vi "Periodic Tasks.vi"(8 "error in (no error)":errorcluster) -> ()   [LabVIEW 2013]
doc: "This VI runs in parallel to other tasks. It can contain as many user-defined periodic loops as you need. These can carry out PID or other sorts of timed response."
uses:
  PnuematicMode.ctl
  <vilib>/Rock Robotics/SystemInterfaces/Utilities/FPGA_UtilitiesLED Source.ctl
  <vilib>/Rock Robotics/SystemInterfaces/Utilities/FPGA_UtilitiesLED State.ctl
  TankDriveAction.ctl
  Example_Code/Ultrasonic/SonarAction.ctl
  AutoAlignMode.ctl
  Example_Code/Gyro/Read Angle Mode.ctl
  Robot Global Data.vi
  <vilib>/Rock Robotics/WPI/Compressor/WPI_CompressorGetSetRefNum.vi
  AutoDistance.vi
panel:
  in  "GyroBrakeScaler":dbl=1.0
  out "Finished":bool=TRUE
  in  "AccelRate":dbl
  out "HandleInputElements":i32
  out "Angle":dbl(knob) scale=0.0..360.0
  out "CurrentAngle":dbl(knob) scale=0.0..360.0
  in  "DesiredAngle":dbl format="%#_13g"
  out "CurrentDistance":dbl(slide)=255.4405658841941 scale=0.0..250.0 scale format="%3d"
  in  "Slowdown":dbl format="%#_13g"
  in  "Brake":dbl format="%#_13g"
  in  "DesiredDistance":dbl format="%#_13g"
  out "Drive loop time":u32
  out "DriveQueueElements":i32
  out "error out":errorcluster
  # "GYRO"
  # "DRIVE"
  # "AUTODISTANCE"
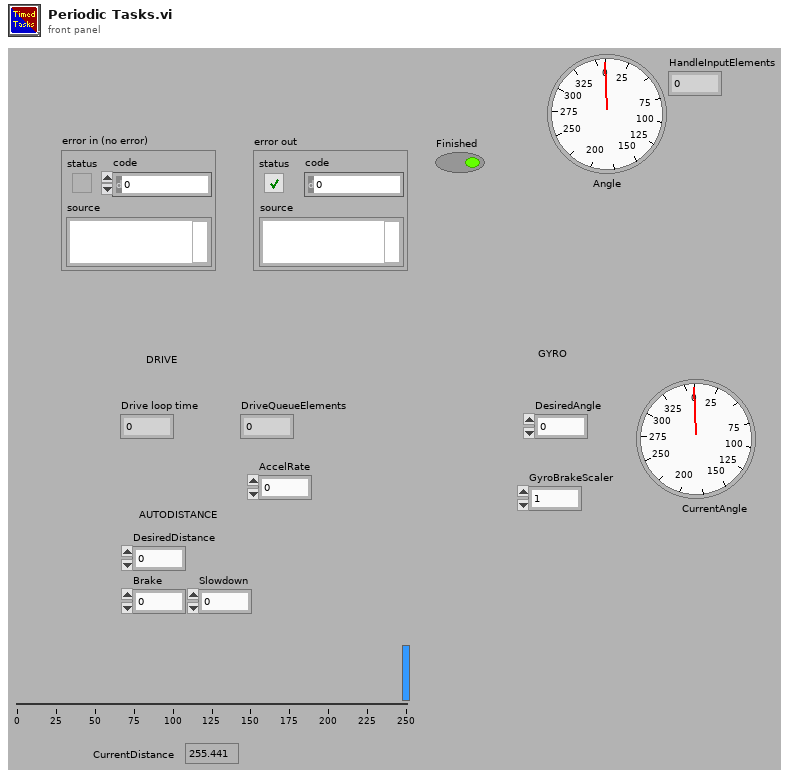
[diagram p1: front panel]
types:
  T1 = typedef "WPI_EncoderDevRef.ctl" = cluster{"DevStatus":errorcluster, "EncoderIndex":T2, "CounterIndex":T3, "DistancePerCount":dbl, "Decoding Type":T4}
  T2 = typedef "FPGA_EncoderIdx.ctl" = enum8{"Enc 0", "Enc 1", "Enc 2", "Enc 3", "Invalid"}
  T3 = typedef "FPGA_CounterCtrSystemIndex.ctl" = enum8{"Ctr 0", "Ctr 1", "Ctr 2", "Ctr 3", "Ctr 4", "Ctr 5", "Ctr 6", "Ctr 7", "Invalid"}
  T4 = typedef "WPI_EncoderType.ctl" = enum16{"1x", "2x", "4x"}
  T5 = typedef "WPI_SolenoidDevRef.ctl" = cluster{"DevStatus":errorcluster, "Solenoid Module":T6, "Forward Solenoid Channel":T7, "Reverse Solenoid Channel":T7}
  T6 = typedef "FPGA_TypedefSolenoidModule.ctl" = enum16{"Solenoid Module 1", "Solenoid Module 2"}
  T7 = typedef "WPI_SolenoidChannel.ctl" = enum8{"Solenoid 1", "Solenoid 2", "Solenoid 3", "Solenoid 4", "Solenoid 5", "Solenoid 6", "Solenoid 7", "Solenoid 8", "Invalid"}
  T8 = typedef "TankDriveAction.ctl" = enum16{"Init", "LinearDrive", "SetValue", "Disable"}
  T9 = typedef "Read Angle Mode.ctl" = enum16{"Init", "ReadAngle", "Disable"}
  T10 = typedef "SonarAction.ctl" = enum16{"Init", "ReadValue", "Disable"}
  T11 = typedef "AutoAlignMode.ctl" = enum16{"Fullspeed", "Linear"}
  T12 = typedef "DriveQueueInstruction.ctl" = cluster{"DriveInstruction":T13, "Subsystem":T14, "Action":T8, "LoopTiming":u32}
  T13 = typedef "DriveInstruction.ctl" = cluster{"cDriveLeft":dbl, "cDriveRight":dbl, "cHalfDrive":bool, "cStraightDrive":bool}
  T14 = typedef "QueueSubsystem.ctl" = enum16{"Drive", "Arm", "Catapult", "Roller"}
  T15 = typedef "TeleopInstruction.ctl" = cluster{"cDriveLeft":dbl, "cDriveRight":dbl, "cHalfDrive":bool, "cStraightDrive":bool, "cSonicShifter":bool}
  T16 = typedef "WPI_CameraDevRef.ctl" = cluster{"Camera Address":string, "CameraStatus":errorcluster, "Acquire Image Notifier":refnum<notifier>}
  T17 = typedef "PnuematicMode.ctl" = enum16{"Init", "SetState", "Disable"}
  T18 = typedef "FPGA_UtilitiesLED State.ctl" = enum16{"Off", "On", "Toggle"}
  T19 = typedef "FPGA_UtilitiesLED Source.ctl" = enum16{"User LED", "FPGA LED"}
  T20 = typedef "WPI_CompressorDevRef.ctl" = cluster{"DevStatus":errorcluster, "DigitalInputDevRef":T21, "RelayDevRef":T24}
  T21 = typedef "WPI_DigitalInputDevRef.ctl" = cluster{"DevStatus":errorcluster, "DIO Channel":T22, "Digital Module":T23}
  T22 = typedef "FPGA_DIOChannel.ctl" = enum8{"DIO 1", "DIO 2", "DIO 3", "DIO 4", "DIO 5", "DIO 6", "DIO 7", "DIO 8", "DIO 9", "DIO 10", "DIO 11", "DIO 12", "DIO 13", "DIO 14", "Invalid"}
  T23 = typedef "FPGA_TypedefDigitalModule.ctl" = enum16{"Digital Module 1", "Digital Module 2"}
  T24 = typedef "WPI_RelayDevRef.ctl" = cluster{"DevStatus":errorcluster, "Relay Channel":T25, "Digital Module":T23, "Relay Direction":T26}
  T25 = typedef "FPGA_DIORelayChannel.ctl" = enum8{"Relay 1", "Relay 2", "Relay 3", "Relay 4", "Relay 5", "Relay 6", "Relay 7", "Relay 8", "Invalid"}
  T26 = typedef "WPI_RelayDirection.ctl" = enum16{"Both directions", "Forward only", "Reverse only"}
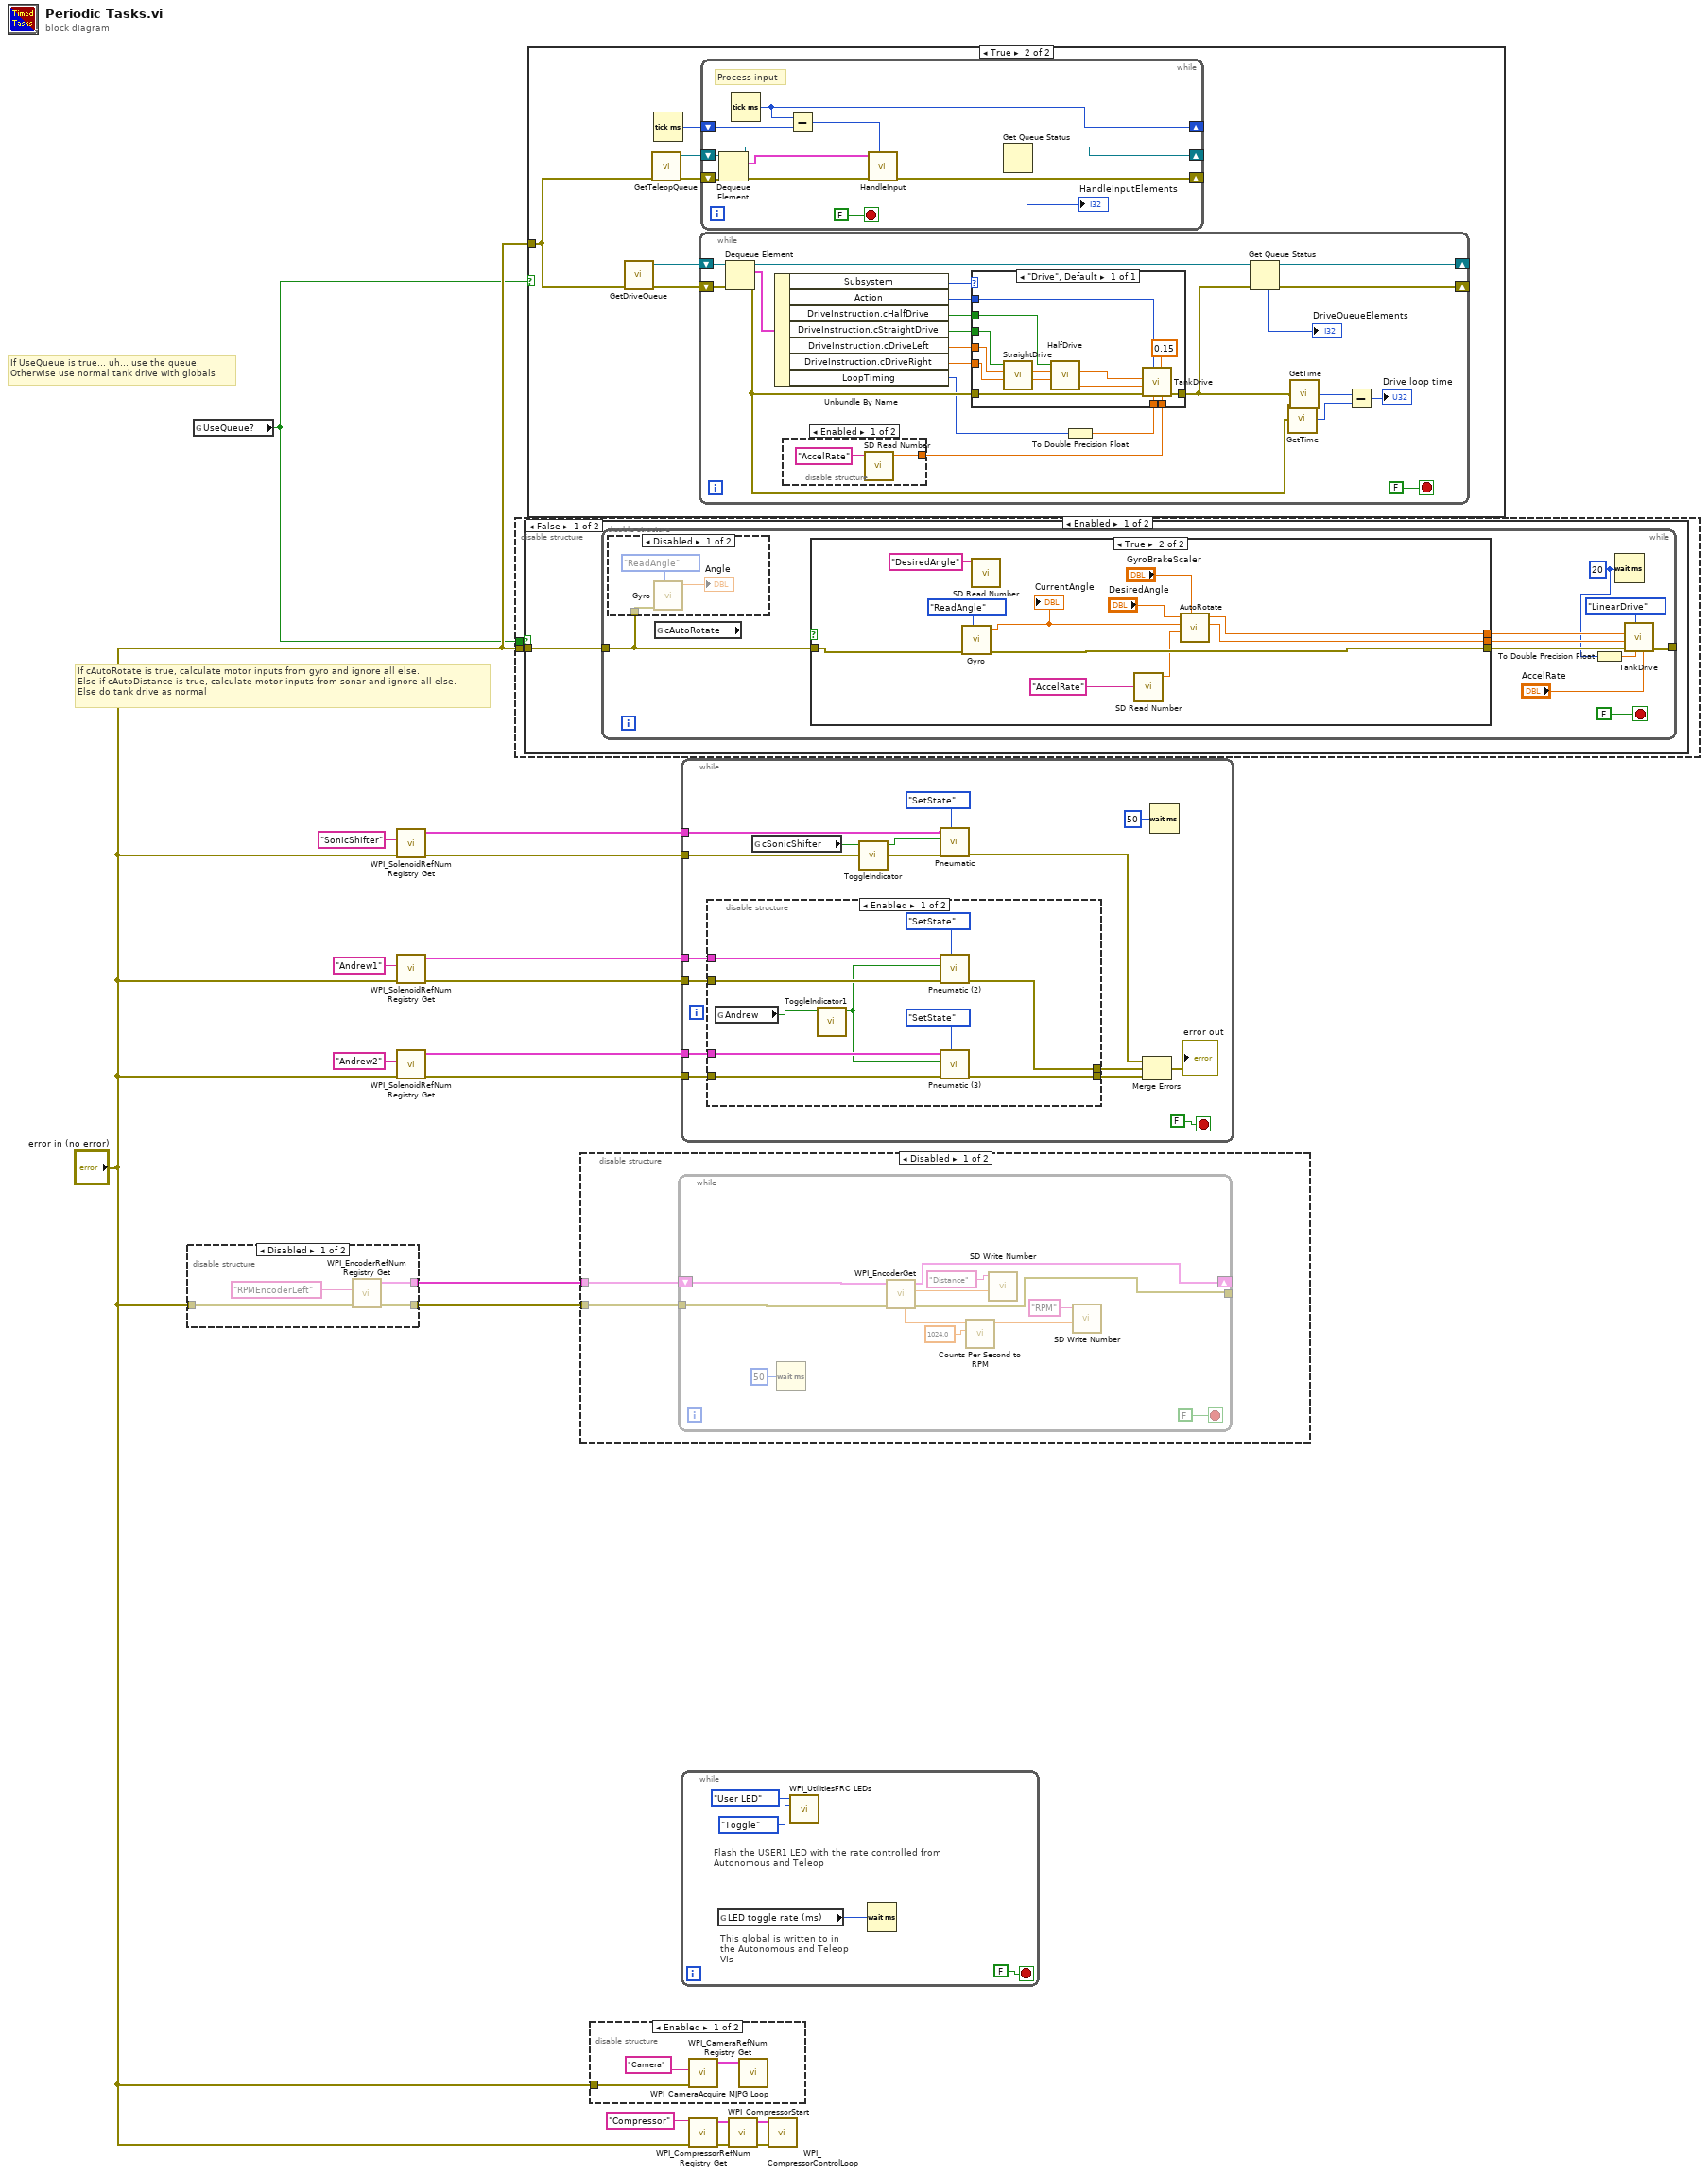
[diagram p0: block diagram]
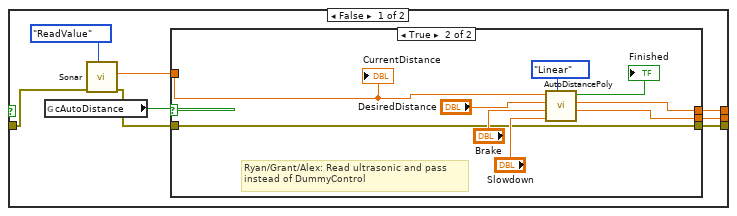
[diagram p3: hidden frame]
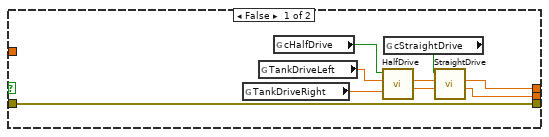
[diagram p4: hidden frame]
diagram:
  # "If UseQueue is true... uh... use the queue.\nOtherwise use normal tank drive with globals"
  # "If cAutoRotate is true, calculate motor inputs from gyro and ignore all else.\nElse if cAutoDistance is true, calculate motor inputs from sonar and ignore all else. \nElse do tank drive as normal"
  n1 = disable-structure shown="Disabled" {
    disable-tunnel: [w21 _] -> w4
    disable-tunnel: [w20 _] -> w3
    disable-tunnel: "error in (no error)" -> [w19 _]
    frame Disabled {
      n2 = call <vilib>:"WPI_EncoderRefNum Registry Get.vi"("error in (no error)"=w19, "refnum name"="RPMEncoderLeft") -> ("error out"=w20:errorcluster, "EncoderDevRef"=w21:T1)  [unwired: 8 in]
    }
    frame Enabled {
    }
  }
  n3 = global read "Robot Global Data.vi" "UseQueue?"() -> (w1:bool)
  n4 = call <vilib>:"WPI_SolenoidRefNum Registry Get.vi"("error in (no error)"="error in (no error)", "refnum name"="SonicShifter") -> ("error out"=w11:errorcluster, "SolenoidDevRef"=w13:T5)  [unwired: 8 in]
  n5 = call <vilib>:"WPI_SolenoidRefNum Registry Get.vi"("error in (no error)"="error in (no error)", "refnum name"="Andrew1") -> ("error out"=w6:errorcluster, "SolenoidDevRef"=w8:T5)  [unwired: 8 in]
  n6 = call <vilib>:"WPI_SolenoidRefNum Registry Get.vi"("error in (no error)"="error in (no error)", "refnum name"="Andrew2") -> ("error out"=w5:errorcluster, "SolenoidDevRef"=w7:T5)  [unwired: 8 in]
  n7 = disable-structure shown="Enabled" {
    disable-tunnel: "error in (no error)" -> [w24 _]
    disable-tunnel: w1 -> [w23 _]
    frame Enabled {
      n8 = case shown="False" w23 {
        tunnel: w24 -> [w25 _]
        frame False {
          n9 = while {
            tunnel: w25 -> [w32]
            tunnel: [w35] -> _
            stop <- FALSE stop-if-true
            w26 = u32 20 ("milliseconds to wait")
            n10 = disable-structure shown="Disabled" {
              disable-tunnel: w32 -> [w39 _]
              frame Disabled {
                n11 = call "Gyro.vi"("Action"=Read_Angle_Mode."ReadAngle", "error in"=w39) -> ("Angle"=→"Angle":dbl)  [unwired: 8 in, 1 out]
              }
              frame Enabled {
              }
            }
            n12 = global read "Robot Global Data.vi" "cAutoRotate"() -> (w33:bool)
            n13 = case shown="True" w33 {
              tunnel: [w47 w70] -> w30
              tunnel: [w46 w71] -> w28
              tunnel: w32 -> [w41 w73]
              tunnel: [w44 w72] -> w29
              frame False {
                n14 = global read "Robot Global Data.vi" "cAutoDistance"() -> (w45:bool)
                n15 = call "Sonar.vi"("Action"=SonarAction."ReadValue", "error in (no error)"=w41) -> ("error out"=w42:errorcluster, "distance"=w43:dbl)  [unwired: 8 in]
                n16 = case shown="True" w45 {
                  tunnel: [w54 w61] -> w47
                  tunnel: [w53 w60] -> w46
                  tunnel: w42 -> [w48 w58]
                  tunnel: [w48 w58] -> w44
                  tunnel: w43 -> [_ w59]
                  frame False {
                    n17 = global read "Robot Global Data.vi" "TankDriveRight"() -> (w51:dbl)
                    n18 = global read "Robot Global Data.vi" "TankDriveLeft"() -> (w52:dbl)
                    n19 = global read "Robot Global Data.vi" "cHalfDrive"() -> (w50:bool)
                    n20 = call "HalfDrive.vi"("RightDrive in"=w51, "LeftDrive in"=w52, "HalfDrive"=w50) -> ("RightDrive out"=w55:dbl, "LeftDrive out"=w56:dbl)  [unwired: 7 in]
                    n21 = global read "Robot Global Data.vi" "cStraightDrive"() -> (w49:bool)
                    n22 = call "StraightDrive.vi"("RightDrive in"=w55, "LeftDrive in"=w56, "StraightDrive"=w49) -> ("RightDrive out"=w53:dbl, "LeftDrive out"=w54:dbl)  [unwired: 7 in]
                  }
                  frame True {
                    # "Ryan/Grant/Alex: Read ultrasonic and pass\ninstead of DummyControl"
                    n23 = call-poly "AutoDistancePoly.vi"("Mode"=AutoAlignMode."Linear", "Slowdown"="Slowdown", "Brake"="Brake", "DesiredDistance"="DesiredDistance", "CurrentDistance"=w59) -> ("TankDriveRight"=w60:dbl, "TankDriveLeft"=w61:dbl, "Finished"=→"Finished":bool)  [unwired: 4 in]
                    "CurrentDistance" <- w59
                  }
                }
              }
              frame True {
                n24 = call "Gyro.vi"("Action"=Read_Angle_Mode."ReadAngle", "error in"=w73) -> ("error out"=w72:errorcluster, "Angle"=w69:dbl)  [unwired: 8 in]
                "CurrentAngle" <- w69
                n25 = call <vilib>:"SD Read Number.vi"("Name"="DesiredAngle") -> ()  [unwired: 8 in, 3 out]
                n26 = call <vilib>:"SD Read Number.vi"("Name"="AccelRate") -> ("Numeric"=w67:dbl)  [unwired: 8 in, 2 out]
                n27 = call "AutoRotate.vi"("BreakScaler"="GyroBrakeScaler", "AccelRate"=w67, "Actual"=w69, "Desired"="DesiredAngle") -> ("Right"=w71:dbl, "Left"=w70:dbl)  [unwired: 5 in]
              }
            }
            n28 = To Double Precision Float(number=w26) -> (double precision float=w27:dbl)
            n29 = Wait (ms)(milliseconds to wait=w26) -> ()  [unwired: 1 out]
            n30 = call "TankDrive.vi"("AccelRate"="AccelRate", "LoopTime"=w27, "DriveAction"=TankDriveAction."LinearDrive" ("Enum"), "error in (no error)"=w29, "RightDesired"=w28, "LeftDesired"=w30) -> ("error out"=w35:errorcluster)  [unwired: 5 in]
          }
        }
        frame True {
        }
      }
    }
    frame Disabled {
    }
  }
  n31 = case shown="True" w1 {
    tunnel: "error in (no error)" -> [_ w78]
    frame False {
    }
    frame True {
      n32 = call "GetDriveQueue.vi"("error in (no error)"=w78) -> ("error out"=w81:errorcluster, "queue out"=w80:refnum<queue>)  [unwired: 9 in]
      n33 = call "GetTeleopQueue.vi"("error in (no error)"=w78) -> ("error out"=w82:errorcluster, "queue out"=w77:refnum<queue>)  [unwired: 9 in]
      n34 = Tick Count (ms)() -> (millisecond timer value=w79:u32)
      n35 = while {
        shift-right: [w88] -> _
        shift-left: w81 -> [w102]
        shift-right: [w90] -> _
        shift-left: w80 -> [w100]
        stop <- FALSE stop-if-true
        n36 = Dequeue Element(queue=w100, error in (no error)=w102) -> (queue out=w99:refnum<queue>, element=w92:T12, error out=w85:errorcluster)  [unwired: 1 in, 1 out]
        n37 = Unbundle By Name(w92) -> ("Subsystem"=w98:T14, "Action"=w97:T8, "DriveInstruction.cHalfDrive"=w96:bool, "DriveInstruction.cStraightDrive"=w95:bool, "DriveInstruction.cDriveLeft"=w94:dbl, "DriveInstruction.cDriveRight"=w93:dbl, "LoopTiming"=w84:u32)
        n38 = disable-structure shown="Enabled" {
          disable-tunnel: [w104 _] -> w101
          frame Enabled {
            n39 = call <vilib>:"SD Read Number.vi"("Name"="AccelRate") -> ("Numeric"=w104:dbl)  [unwired: 8 in, 2 out]
          }
          frame Disabled {
          }
        }
        n40 = To Double Precision Float(number=w84) -> (double precision float=w91:dbl)
        n41 = case shown="\"Drive\", Default" w98 {
          tunnel: w85 -> [w115]
          tunnel: [w114] -> w88
          tunnel: w101 -> [w113]
          tunnel: w97 -> [w112]
          tunnel: w96 -> [w110]
          tunnel: w95 -> [w111]
          tunnel: w94 -> [w109]
          tunnel: w93 -> [w108]
          tunnel: w91 -> [w107]
          frame "Drive", Default {
            n42 = call "StraightDrive.vi"("RightDrive in"=w108, "LeftDrive in"=w109, "StraightDrive"=w111) -> ("RightDrive out"=w118:dbl, "LeftDrive out"=w119:dbl)  [unwired: 7 in]
            n43 = call "HalfDrive.vi"("RightDrive in"=w118, "LeftDrive in"=w119, "HalfDrive"=w110) -> ("RightDrive out"=w116:dbl, "LeftDrive out"=w117:dbl)  [unwired: 7 in]
            n44 = call "TankDrive.vi"("AccelRate"=w113, "Cutoff"=0.15, "LoopTime"=w107, "DriveAction"=w112, "error in (no error)"=w115, "RightDesired"=w116, "LeftDesired"=w117) -> ("error out"=w114:errorcluster)  [unwired: 4 in]
          }
        }
        n45 = Get Queue Status(queue=w99) -> (queue out=w90:refnum<queue>, # elements in queue=→"DriveQueueElements":i32)  [unwired: 2 in, 6 out]
        n46 = call "GetTime.vi"("error in"=w85) -> ("Time"=w86:u32)
        n47 = call "GetTime.vi"("error in"=w88) -> ("Time"=w87:u32)
        n48 = Subtract(x=w87, y=w86) -> (x-y=→"Drive loop time":u32)
      }
      n49 = while {
        shift-right: [w129] -> _
        shift-left: w82 -> [w131]
        shift-right: [w127] -> _
        shift-left: w79 -> [w128]
        shift-right: [w121] -> _
        shift-left: w77 -> [w124]
        stop <- FALSE stop-if-true
        # "Process input"
        n50 = Dequeue Element(queue=w124, error in (no error)=w131) -> (queue out=w122:refnum<queue>, element=w123:T15, error out=w130:errorcluster)  [unwired: 1 in, 1 out]
        n51 = Tick Count (ms)() -> (millisecond timer value=w127:u32)
        n52 = Subtract(x=w127, y=w128) -> (x-y=w126:u32)
        n53 = call "HandleInput.vi"("LoopTiming"=w126, "error in (no error)"=w130, "TeleopInstruction"=w123) -> ("error out"=w129:errorcluster)  [unwired: 8 in]
        n54 = Get Queue Status(queue=w122) -> (queue out=w121:refnum<queue>, # elements in queue=→"HandleInputElements":i32)  [unwired: 2 in, 6 out]
      }
    }
  }
  n55 = disable-structure shown="Disabled" {
    disable-tunnel: w4 -> [w133 _]
    disable-tunnel: w3 -> [w132 _]
    frame Disabled {
      n56 = while {
        tunnel: w132 -> [w142]
        shift-right: [w141] -> _
        shift-left: w133 -> [w143]
        tunnel: [w134] -> _
        stop <- FALSE stop-if-true
        n57 = Wait (ms)(milliseconds to wait=u32 50) -> ()  [unwired: 1 out]
        n58 = call <vilib>:"WPI_EncoderGet.vi"("error in (no error)"=w142, "EncoderDevRef"=w143) -> ("error out"=w134:errorcluster, "Distance"=w136:dbl, "EncoderDevRef"=w141:T1, "Rate"=w140:dbl)  [unwired: 4 in, 2 out]
        n59 = call "Counts Per Second to RPM.vi"("Counts/Rev"=1024.0, "Counts/Second"=w140) -> ("RPM"=w138:dbl)  [unwired: 9 in]
        n60 = call <vilib>:"SD Write Number.vi"("Numeric"=w136, "Name"="Distance") -> ()  [unwired: 8 in, 2 out]
        n61 = call <vilib>:"SD Write Number.vi"("Numeric"=w138, "Name"="RPM") -> ()  [unwired: 8 in, 2 out]
      }
    }
    frame Enabled {
    }
  }
  n62 = disable-structure shown="Enabled" {
    disable-tunnel: "error in (no error)" -> [w146 _]
    frame Enabled {
      n63 = call <vilib>:"WPI_CameraRefNum Registry Get.vi"("error in (no error)"=w146, "refnum name"="Camera") -> ("CameraDevRef"=w147:T16)  [unwired: 8 in, 1 out]
      n64 = call <vilib>:"WPI_CameraAcquire MJPG Loop.vi"("CameraDevRef"=w147) -> ()  [unwired: 11 in]
    }
    frame Disabled {
    }
  }
  n65 = while {
    tunnel: w13 -> [w161]
    tunnel: w11 -> [w162]
    tunnel: w8 -> [w157]
    tunnel: w7 -> [w156]
    tunnel: w6 -> [w159]
    tunnel: w5 -> [w155]
    stop <- FALSE stop-if-true
    n66 = disable-structure shown="Enabled" {
      disable-tunnel: w159 -> [w173 _]
      disable-tunnel: [w172 _] -> w158
      disable-tunnel: w157 -> [w171 _]
      disable-tunnel: w156 -> [w169 _]
      disable-tunnel: w155 -> [w168 _]
      disable-tunnel: [w167 _] -> w154
      frame Enabled {
        n67 = global read "Robot Global Data.vi" "Andrew"() -> (w165:bool)
        n68 = call "ToggleIndicator1.vi"("cSonicShifter"=w165) -> ("Actuate?"=w164:bool)  [unwired: 10 in]
        n69 = call "Pneumatic (2).vi"("Mode"=PnuematicMode."SetState", "error in (no error)"=w173, "State"=w164, "SolenoidDevRef"=w171) -> ("error out"=w172:errorcluster)  [unwired: 7 in]
        n70 = call "Pneumatic (3).vi"("Mode"=PnuematicMode."SetState", "error in (no error)"=w168, "State"=w164, "SolenoidDevRef"=w169) -> ("error out"=w167:errorcluster)  [unwired: 7 in]
      }
      frame Disabled {
      }
    }
    n71 = global read "Robot Global Data.vi" "cSonicShifter"() -> (w153:bool)
    n72 = call "ToggleIndicator.vi"("cSonicShifter"=w153) -> ("Actuate?"=w152:bool)  [unwired: 10 in]
    n73 = call "Pneumatic.vi"("Mode"=PnuematicMode."SetState", "error in (no error)"=w162, "State"=w152, "SolenoidDevRef"=w161) -> ("error out"=w149:errorcluster)  [unwired: 7 in]
    n74 = Merge Errors(w149, w158, w154) -> (→"error out":errorcluster)
    n75 = Wait (ms)(milliseconds to wait=u32 50) -> ()  [unwired: 1 out]
  }
  n76 = while {
    stop <- FALSE stop-if-true
    # "This global is written to in the Autonomous and Teleop VIs"
    # "Flash the USER1 LED with the rate controlled from Autonomous and Teleop"
    n77 = global read "Robot Global Data.vi" "LED toggle rate (ms)"() -> (w174:u32)
    n78 = call <vilib>:"WPI_UtilitiesFRC LEDs.vi"("State"=FPGA_UtilitiesLED_State."Toggle", "LED Type"=FPGA_UtilitiesLED_Source."User LED") -> ()  [unwired: 1 in, 9 out]
    n79 = Wait (ms)(milliseconds to wait=w174) -> ()  [unwired: 1 out]
  }
  n80 = call <vilib>:"WPI_CompressorRefNum Registry Get.vi"("error in (no error)"="error in (no error)", "refnum name"="Compressor") -> ("error out"=w15:errorcluster, "CompressorDevRef"=w18:T20)  [unwired: 8 in]
  n81 = call <vilib>:"WPI_CompressorStart.vi"("error in (no error)"=w15, "CompressorDevRef"=w18) -> ("error out"=w12:errorcluster, "CompressorDevRef"=w17:T20)  [unwired: 8 in]
  n82 = call <vilib>:"WPI_CompressorControlLoop.vi"("error in (no error)"=w12, "CompressorDevRef"=w17) -> ()  [unwired: 10 in]
